vi "Update Holt State.vi"(8 "error in (no error)":errorcluster, 11 "1553 Component in":refnum<class "1553 Component.lvclass">) -> (0 "error out":errorcluster, 3 "1553 Component out":refnum<class "1553 Component.lvclass">)   [LabVIEW 2020, in "BCI-1553 API.lvlib" / "1553 Component.lvclass"]
doc: "Updates the 1553 Session hardware with the current data stored in the component Virtual Memory."
uses:
  1553 Component.lvclass
  1553 Component.lvclass/1553 Component.ctl
  Dependencies/FPGA Interface/FPGA Interface.lvclass
  Dependencies/Virtual Memory Unit/Virtual Memory Unit.lvclass
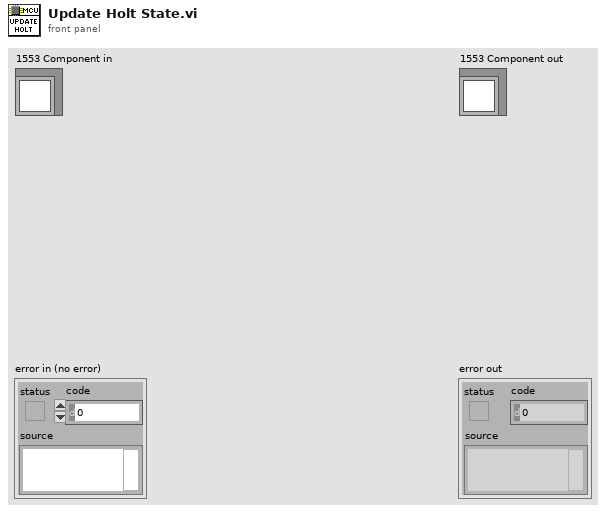
[diagram p1: front panel]
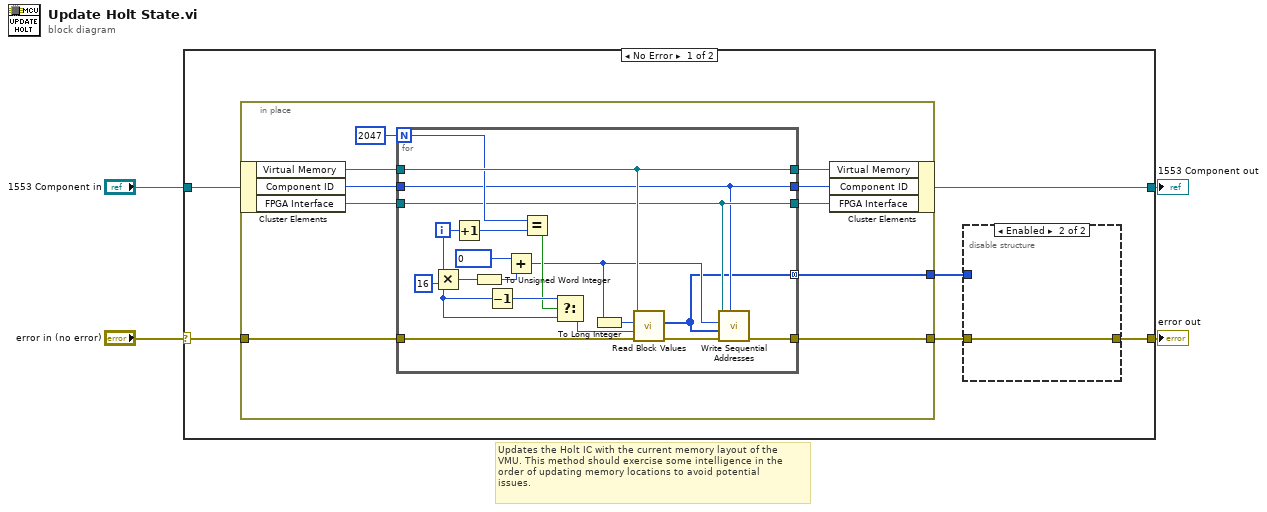
[diagram p0: block diagram]
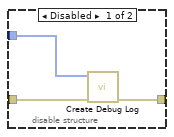
[diagram p2: hidden frame]
diagram:
  # "Updates the Holt IC with the current memory layout of the\nVMU. This method should exercise some intelligence in the\norder of updating memory locations to avoid potential\nissues."
  n1 = case shown="No Error" "error in (no error)" {
    selector: "error in (no error)" -> [w10 w45]
    tunnel: [w7 w45] -> w3
    tunnel: [w8 w44] -> w1
    tunnel: "1553 Component in" -> [w9 w44]
    frame No Error {
      n2 = in-place {
        in-place-border: w10 -> [w20]
        in-place-border: [w13] -> w6
        in-place-border: [w11] -> w5
        n3 = in-place-cluster #1(w9) -> ("Virtual Memory"=w18:refnum<class "Virtual Memory Unit.lvclass">, "Component ID"=w17:u8, "FPGA Interface"=w16:refnum<class "FPGA Interface.lvclass">)
        n4 = for {
          N: 2047 -> [w31]
          tunnel: w20 -> [w35]
          tunnel: w16 -> [w26]
          tunnel: w17 -> [w25]
          tunnel: [w25] -> w12
          tunnel: [w26] -> w14
          tunnel: w18 -> [w36]
          tunnel: [w36] -> w15
          tunnel: [w22] -> w13
          tunnel: [w21] -> w11 mode=concatenating
          i -> [w32]
          w27 = 16 ("y")
          n5 = Multiply(x=w32, y=w27) -> (x*y=w39:i32)
          n6 = Increment(x=w32) -> (x+1=w30:i32)
          n7 = To Unsigned Word Integer(number=w39) -> (unsigned 16bit integer=w38:u16)
          n8 = Decrement(x=w27) -> (x-1=w29:i32)
          n9 = Add(x=u16 0 ("Address"), y=w38) -> (x+y=w24:u16)
          n10 = Equal?(x=w31, y=w30) -> (x = y?=w28:bool)
          n11 = Select(t=w29, s=w28, f=w27) -> (s? t:f=w23:i32)
          n12 = To Long Integer(number=w24) -> (32bit integer=w33:i32)
          n13 = call "Read Block Values.vi"("error in (no error)"=w35, "Read Length"=w23, "Start Index"=w33, "Virtual Memory Unit in"=w36) -> ("error out"=w34:errorcluster, "Read Block"=w21:u16[])  [unwired: 6 in]
          n14 = call-dynamic "Write Sequential Addresses.vi"("Target IC (1-8)"=w25, "error in (no error)"=w34, "Data"=w21, "Starting Address"=w24, "FPGA Interface in"=w26) -> ("error out"=w22:errorcluster)  [unwired: 6 in]
        }
        n15 = in-place-cluster #1("Virtual Memory"=w15, "Component ID"=w12, "FPGA Interface"=w14) -> (w8:refnum<class "1553 Component.lvclass">)
      }
      n16 = disable-structure shown="Enabled" {
        disable-tunnel: [w40 w43] -> w7
        disable-tunnel: w6 -> [w41 w43]
        disable-tunnel: w5 -> [w42 _]
        frame Disabled {
          n17 = call "Create Debug Log.vi"("error in (no error)"=w41, "Pre-Push data"=w42) -> ("error out"=w40:errorcluster)  [unwired: 9 in]
        }
        frame Enabled {
        }
      }
    }
    frame Error {
    }
  }
  "error out" <- w3
  "1553 Component out" <- w1
